vi "Get Test Time.vi"(8 "error in (no error)":errorcluster, 10 "loop iteration":i32, 11 "start time in":timestamp) -> (0 "error out":errorcluster, 2 "current time":dbl, 3 "start time out":timestamp)   [LabVIEW 2020]
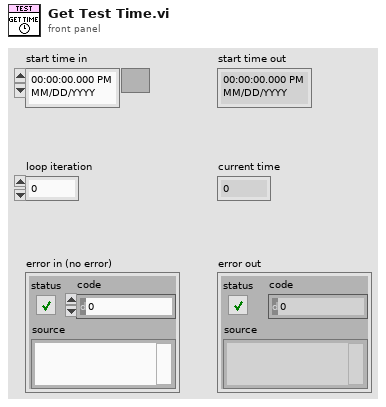
[diagram p1: front panel]
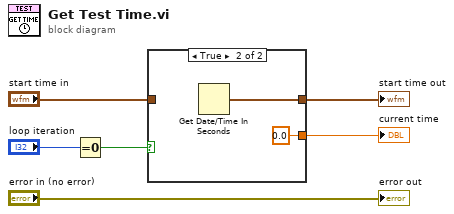
[diagram p0: block diagram]
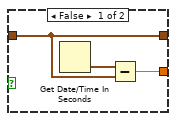
[diagram p2: hidden frame]
diagram:
  n1 = Equal To 0?(x="loop iteration") -> (x = 0?=w4:bool)
  n2 = case shown="True" w4 {
    tunnel: "start time in" -> [w7 _]
    tunnel: [w7 w11] -> w1
    tunnel: [w9 0.0] -> w2
    frame False {
      n3 = Get Date/Time In Seconds() -> (seconds since 1Jan1904=w8:timestamp)
      n4 = Subtract(x=w8, y=w7) -> (x-y=w9:dbl)
    }
    frame True {
      n5 = Get Date/Time In Seconds() -> (seconds since 1Jan1904=w11:timestamp)
    }
  }
  "current time" <- w2
  "start time out" <- w1
  "error out" <- "error in (no error)"
